vi "GVDA Gas Viscosity of Dry Air (kg to m to s).vi"(1 "Tceg\nGas Temperature":dbl[unit]=10.0 min=10.0 max=95.0) -> (0 "Gas Viscosity\nof Dry Air":dbl[unit])   [LabVIEW 2018]
panel:
  out "Temprature Of Input Air\nKelvin Degree":dbl[unit](slide) scale=273.0..373.0
  out "Tk":dbl[unit]
  out "Temprature Of Input Air\nCentigrade Degree":dbl[unit](slide) scale=0.0..100.0
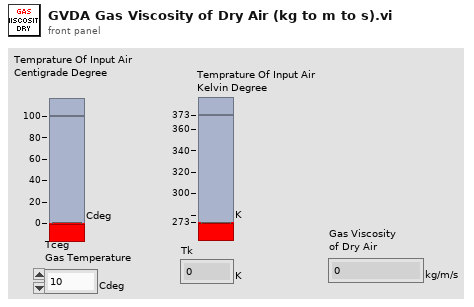
[diagram p1: front panel]
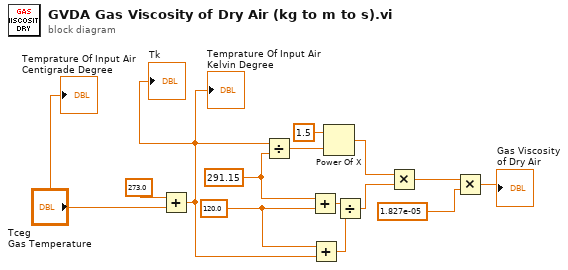
[diagram p0: block diagram]
diagram:
  w8 = dbl[unit] 120.0 ("y")
  w9 = dbl[unit] 291.15 ("y")
  n1 = Add(x=dbl[unit] 273.0 ("y"), y="Tceg\nGas Temperature") -> (x+y=w2:dbl[unit])
  "Tk" <- w2
  "Temprature Of Input Air\nKelvin Degree" <- w2
  n2 = Divide(x=w2, y=w9) -> (x/y=w14:dbl)
  n3 = Add(x=w9, y=w8) -> (x+y=w11:dbl[unit])
  n4 = Add(x=w8, y=w2) -> (x+y=w10:dbl[unit])
  n5 = Power Of X(1:w14, 2:1.5 ("y")) -> (0:w3:dbl)
  n6 = Divide(x=w11, y=w10) -> (x/y=w12:dbl)
  n7 = Multiply(x=w3, y=w12) -> (x*y=w7:dbl)
  n8 = Multiply(x=w7, y=dbl[unit] 1.827e-05) -> (x*y=→"Gas Viscosity\nof Dry Air":dbl[unit])
  "Temprature Of Input Air\nCentigrade Degree" <- "Tceg\nGas Temperature"
